vi "AddNode.vi"(8 "error in":errorcluster, 9 "node in":refnum<class "NISE_CEF_Node.lvclass">, 10 "parent node ID":string) -> (0 "error out":errorcluster, 2 "summary":T1[](array[typedef]))   [LabVIEW 2013, in "NISE_CEF_TreeControl.lvlib"]
doc: "This Vi adds a new node to the Parent Node ID"
uses:
  NISE_CEF_TreeControl.lvlib
  Node/Summary.ctl
  Node/NISE_CEF_Node.lvclass
  Node/NISE_CEF_Node.lvclass/NISE_CEF_Node.ctl
  Node/ReadChildren.vi
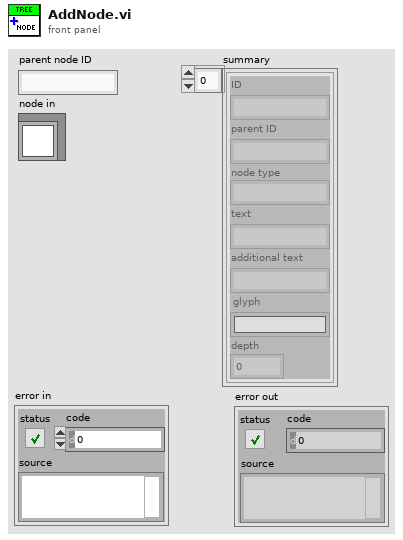
[diagram p1: front panel]
types:
  T1 = typedef "NISE_CEF_Node.lvclass/Summary.ctl" = cluster{"ID":string, "parent ID":string, "node type":string, "text":string, "additional text":string, "glyph":string, "depth":i32}
  T2 = typedef "NISE_CEF_Node.lvclass/NodeRef.ctl" = refnum<data-value>
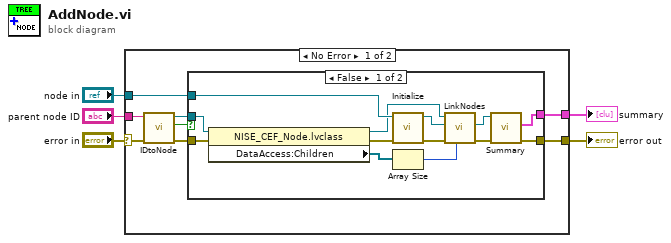
[diagram p0: block diagram]
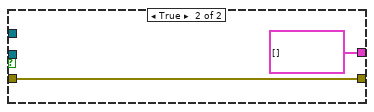
[diagram p2: hidden frame]
diagram:
  n1 = case shown="No Error" "error in" {
    selector: "error in" -> [w8 w29]
    tunnel: "parent node ID" -> [w13 _]
    tunnel: [w11 _] -> w3
    tunnel: [w10 w29] -> w2
    tunnel: "node in" -> [w9 _]
    frame No Error {
      n2 = call "IDtoNode.vi"("error in"=w8, "ID"=w13) -> ("error out"=w7:errorcluster, "invalid Id"=w6:bool, "node ref"=w12:T2)  [unwired: 7 in]
      n3 = case shown="False" w6 {
        tunnel: w12 -> [w19 _]
        tunnel: [w26 T1[] [] ("summary")] -> w11
        tunnel: [w25 w28] -> w10
        tunnel: w9 -> [w22 _]
        tunnel: w7 -> [w15 w28]
        frame False {
          n4 = property class="NISE_CEF_Node.lvclass"(reference=w19, error in=w15) -> (reference out=w18:T2, error out=w14:errorcluster, "DataAccess:Children"=w17:T2[])
          n5 = call-dynamic "Initialize.vi"("error in"=w14, "node in"=w22) -> ("error out"=w20:errorcluster, "data value reference"=w21:T2)  [unwired: 7 in, 1 out]
          n6 = Array Size(array=w17) -> (size(s)=w16:i32)
          n7 = call "LinkNodes.vi"("index"=w16, "error in"=w20, "child in"=w21, "parent in"=w18) -> ("error out"=w24:errorcluster, "child out"=w23:T2)  [unwired: 5 in, 1 out]
          n8 = call "Summary.vi"("error in"=w24, "node self ref"=w23) -> ("error out"=w25:errorcluster, "summary"=w26:T1[])  [unwired: 8 in]
        }
        frame True {
        }
      }
    }
    frame Error {
    }
  }
  "error out" <- w2
  "summary" <- w3
